vi "End RouteGuide RecordRoute.vi"(7 "Occurrence":enum16{"With Occurrence", "Without Occurrence"}(ring), 8 "error in":errorcluster, 11 "Call ID in":T3) -> (0 "error out":errorcluster, 1 "errorDetails":T1, 2 "Response Data":T2)   [LabVIEW 2019, in "route_guide_client.lvlib"]
uses:
  route_guide_client.lvlib
  <vilib>/gRPC/LabVIEW gRPC Library/Shared/grpcId.ctl
  RPC Messages/routeguide_RouteSummary.ctl
  <vilib>/gRPC/LabVIEW gRPC Library/Shared/Any.ctl
  RPC Messages/routeguide_RouteSummary_Flat.ctl
  2435b599-b0f7-48e4-804e-62ee509d3e35.vi
  <vilib>/gRPC/LabVIEW gRPC Library/Shared/TranslateGrpcError.vi
  <vilib>/gRPC/LabVIEW gRPC Library/Shared/Wait On Occurence.vi
  <vilib>/gRPC/LabVIEW gRPC Library/Server API/Server/Get Server DLL Path.vi
  <vilib>/Utility/error.llb/Error Cluster From Error Code.vi
  <vilib>/gRPC/LabVIEW gRPC Library/grpc-lvsupport-release.lvlib
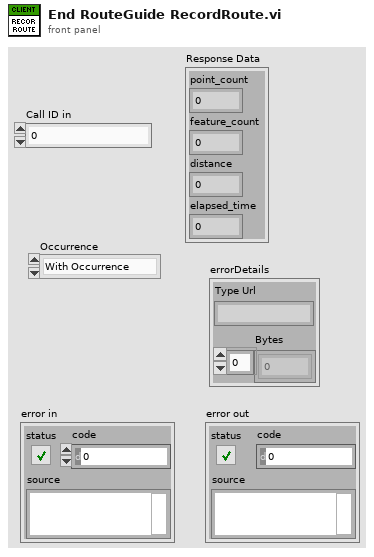
[diagram p1: front panel]
types:
  T1 = typedef "grpc-lvsupport-release.lvlib/Any.ctl" = cluster{"Type Url":string, "Bytes":u8[]}
  T2 = typedef "route_guide_client.lvlib/routeguide_RouteSummary.ctl" = cluster{"point_count":i32, "feature_count":i32, "distance":i32, "elapsed_time":i32}
  T3 = typedef "grpc-lvsupport-release.lvlib/grpcId.ctl" = u64
  T4 = typedef "route_guide_client.lvlib/routeguide_RouteSummary_Flat.ctl" = cluster{"point_count":i32, "feature_count":i32, "distance":i32, "elapsed_time":i32}
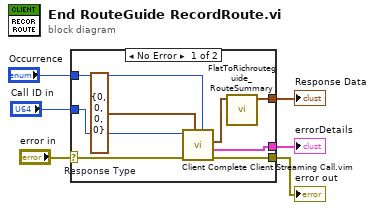
[diagram p0: block diagram]
diagram:
  n1 = case shown="No Error" "error in" {
    selector: "error in" -> [w14 w15]
    tunnel: [w13 w15] -> w5
    tunnel: "Call ID in" -> [w12 _]
    tunnel: [w8 _] -> w3
    tunnel: [w10 _] -> w2
    tunnel: "Occurrence" -> [w7 _]
    frame No Error {
      w11 = T4 {"point_count"=0, "feature_count"=0, "distance"=0, "elapsed_time"=0}  # Response Type
      n2 = call "Client Complete Client Streaming Call.vim"("Occurrence"=w7, "Response Type"=w11, "error in"=w14, "Call ID in"=w12) -> ("error out"=w13:errorcluster, "errorDetails"=w10:T1, "Response Data"=w9:T4)  [unwired: 5 in]
      n3 = call "FlatToRichrouteguide_RouteSummary.vi"("InputCluster"=w9) -> ("OutputCluster"=w8:T2)  [unwired: 10 in]
    }
    frame Error {
    }
  }
  "error out" <- w5
  "Response Data" <- w3
  "errorDetails" <- w2
